vi "HW_GEN - Check VCH[] Formula.vi"(11 "UsedModuCFG":T1[](array[typedef])) -> (3 "VarList":cluster{"Tag":string[], "Alias":string[]})   [LabVIEW 2016]
uses:
  Ctrls/HardWare _ Module Configuration.ctl
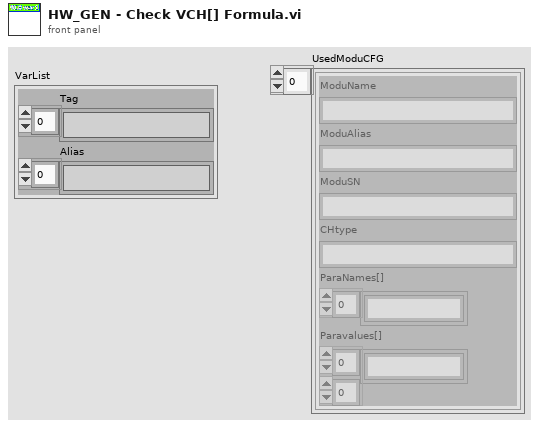
[diagram p1: front panel]
types:
  T1 = typedef "HardWare _ Module Configuration.ctl" = cluster{"ModuName":string, "ModuAlias":string, "ModuSN":string, "CHtype":string, "ParaNames[]":string[], "Paravalues[]":string[][]}
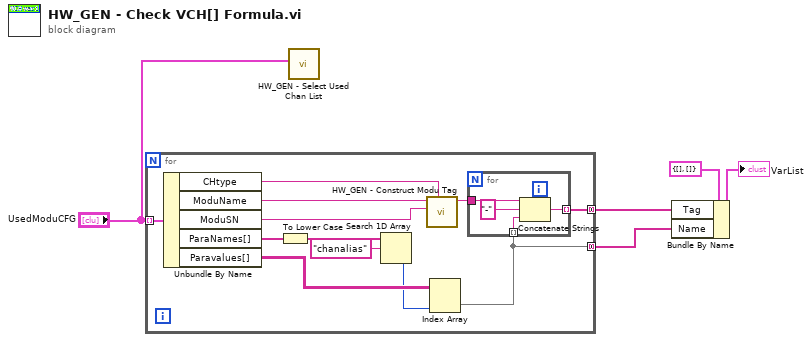
[diagram p0: block diagram]
diagram:
  n1 = for {
    tunnel: [w16] -> w4 mode=concatenating
    tunnel: "UsedModuCFG" -> [w17] mode=indexing
    tunnel: [w6] -> w2 mode=concatenating
    n2 = Unbundle By Name(w17) -> ("CHtype"=w13:string, "ModuName"=w15:string, "ModuSN"=w14:string, "ParaNames[]"=w11:string[], "Paravalues[]"=w8:string[][])
    n3 = To Lower Case(string=w11) -> (all lower case string=w9:string[])
    n4 = Search 1D Array(1D array=w9, element="chanalias") -> (index of element=w7:i32)  [unwired: 1 in]
    n5 = call "HW_GEN - Construct Modu Tag.vi"("ChanType"=w13, "ModSN"=w14, "ModName"=w15) -> ("String"=w12:string)  [unwired: 8 in]
    n6 = Index Array(array=w8, index (col)=w7) -> (element=w6:string[])  [unwired: 1 in]
    n7 = for {
      tunnel: w12 -> [w21]
      tunnel: [w19] -> w16 mode=indexing
      tunnel: w6 -> [w18] mode=indexing
      n8 = Concatenate Strings(w21, "-" ("string"), w18) -> (w19:string)
    }
  }
  n9 = call "HW_GEN - Select Used Chan List.vi"("Cfg in"="UsedModuCFG") -> ()  [unwired: 9 in, 2 out]
  n10 = Bundle By Name(cluster=cluster{"Tag":string[], "Name":string[]} {"Tag"=[], "Name"=[]} ("VarList"), "Tag"=w4, "Name"=w2) -> (→"VarList":cluster{"Tag":string[], "Name":string[]})
